vi "endeffector.vi"() -> ()   [LabVIEW 2018]
uses:
  <vilib>/MediaMongrels Ltd/WebSockets/WebSockets/WebSocket Client/WebSocket Client.lvclass
  D:/software_setup/National Instruments/LabVIEW 2018/vi.lib/MediaMongrels Ltd/WebSockets/WebSockets/WebSocket/WebSocket.lvclass
panel:
  out "suction_isOn":bool
  out "suction_isEnabled":bool
  out "zOffset":dbl
  out "yOffset":dbl
  out "xOffset":dbl
  out "laser_isOn":bool
  out "laser_isEnabled":bool
  out "gripper_isOn":bool
  out "gripper_isEnabled":bool
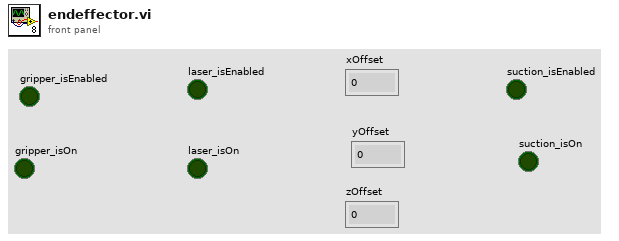
[diagram p1: front panel]
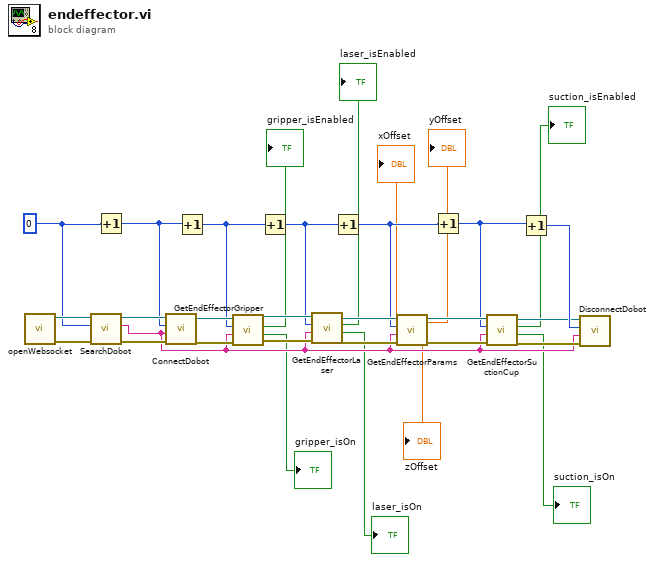
[diagram p0: block diagram]
diagram:
  w27 = 0 ("id")
  n1 = call <vilib>:"openWebsocket.vi"() -> ("error out"=w29:errorcluster, "WebSocket Client out"=w31:refnum<class "WebSocket Client.lvclass">)  [unwired: 10 in]
  n2 = call <vilib>:"SearchDobot.vi"("error in (no error)"=w29, "id"=w27, "WebSocket in"=w31) -> ("error out"=w28:errorcluster, "portName"=w10:string, "WebSocket out"=w30:refnum<class "WebSocket Client.lvclass">)  [unwired: 6 in]
  n3 = Increment(x=w27) -> (x+1=w26:i32)
  n4 = call <vilib>:"ConnectDobot.vi"("error in (no error)"=w28, "portName"=w10, "id"=w26, "WebSocket in"=w30) -> ("error out"=w15:errorcluster, "WebSocket out"=w24:refnum<class "WebSocket Client.lvclass">)  [unwired: 5 in, 1 out]
  n5 = Increment(x=w26) -> (x+1=w14:i32)
  n6 = call <vilib>:"GetEndEffectorGripper.vi"("error in (no error)"=w15, "portName"=w10, "id"=w14, "WebSocket in"=w24) -> ("error out"=w16:errorcluster, "isOn"=→"gripper_isOn":bool, "isEnabled"=→"gripper_isEnabled":bool, "WebSocket out"=w23:refnum<class "WebSocket Client.lvclass">)  [unwired: 4 in]
  n7 = Increment(x=w14) -> (x+1=w13:i32)
  n8 = call <vilib>:"GetEndEffectorLaser.vi"("error in (no error)"=w16, "portName"=w10, "id"=w13, "WebSocket in"=w23) -> ("error out"=w17:errorcluster, "isOn"=→"laser_isOn":bool, "isEnabled"=→"laser_isEnabled":bool, "WebSocket out"=w22:refnum<class "WebSocket Client.lvclass">)  [unwired: 4 in]
  n9 = Increment(x=w13) -> (x+1=w12:i32)
  n10 = call <vilib>:"GetEndEffectorParams.vi"("error in (no error)"=w17, "portName"=w10, "id"=w12, "WebSocket in"=w22) -> ("error out"=w18:errorcluster, "WebSocket out"=w21:refnum<class "WebSocket Client.lvclass">, "yOffset"=→"yOffset":dbl, "zOffset"=→"zOffset":dbl, "xOffset"=→"xOffset":dbl)  [unwired: 3 in]
  n11 = Increment(x=w12) -> (x+1=w11:i32)
  n12 = call <vilib>:"GetEndEffectorSuctionCup.vi"("error in (no error)"=w18, "portName"=w10, "id"=w11, "WebSocket in"=w21) -> ("error out"=w19:errorcluster, "isOn"=→"suction_isOn":bool, "isEnabled"=→"suction_isEnabled":bool, "WebSocket out"=w20:refnum<class "WebSocket Client.lvclass">)  [unwired: 4 in]
  n13 = Increment(x=w11) -> (x+1=w25:i32)
  n14 = call <vilib>:"DisconnectDobot.vi"("error in (no error)"=w19, "portName"=w10, "id"=w25, "WebSocket in"=w20) -> ()  [unwired: 5 in, 3 out]
